vi "试剂余量显示UI.vi"() -> ()   [LabVIEW 2016, in "斯坦道总磷.lvlib"]
uses:
  <vilib>/Utility/miscctls.llb/LVPointTypeDef.ctl
panel:
  in  "余量 14":string
  in  "余量 13":string
  in  "余量 12":string
  in  "余量 11":string
  in  "余量 10":string
  in  "余量 9":string
  in  "余量 8":string
  in  "余量 7":string
  in  "余量 6":string
  in  "余量 5":string
  in  "余量 4":string
  in  "余量 3":string
  in  "余量 2":string
  in  "余量":string
  in  "关闭":bool
  in  "全部重置":bool
  in  "试剂容量设置":bool
  in  "试剂名称设置":bool
  in  "重置 14":bool
  out "试剂 14":dbl(slide) caption="V9-2.试剂14" scale=0.0..100.0 scale format="%#_f %%"
  in  "重置 13":bool
  out "试剂 13":dbl(slide) caption="V9-1.试剂13" scale=0.0..100.0 scale format="%#_f %%"
  in  "重置 12":bool
  out "试剂 12":dbl(slide) caption="V12.试剂12" scale=0.0..100.0 scale format="%#_f %%"
  in  "重置 11":bool
  out "试剂 11":dbl(slide) caption="V11.试剂11" scale=0.0..100.0 scale format="%#_f %%"
  in  "重置 10":bool
  out "试剂 10":dbl(slide) caption="V10.试剂10" scale=0.0..100.0 scale format="%#_f %%"
  in  "重置 9":bool
  out "试剂 9":dbl(slide) caption="V9.试剂9" scale=0.0..100.0 scale format="%#_f %%"
  in  "重置 8":bool
  out "试剂 8":dbl(slide) caption="V8.试剂8" scale=0.0..100.0 scale format="%#_f %%"
  in  "重置 7":bool
  out "试剂 7":dbl(slide) caption="V7.试剂7" scale=0.0..100.0 scale format="%#_f %%"
  in  "重置 6":bool
  out "试剂 6":dbl(slide) caption="V6.试剂6" scale=0.0..100.0 scale format="%#_f %%"
  in  "重置 5":bool
  out "试剂 5":dbl(slide) caption="V5.试剂5" scale=0.0..100.0 scale format="%#_f %%"
  in  "重置 4":bool
  out "试剂 4":dbl(slide) caption="V4.试剂4" scale=0.0..100.0 scale format="%#_f %%"
  in  "重置 3":bool
  out "试剂 3":dbl(slide) caption="V3.试剂3" scale=0.0..100.0 scale format="%#_f %%"
  in  "重置 2":bool
  out "试剂 2":dbl(slide) caption="V2.试剂2" scale=0.0..100.0 scale format="%#_f %%"
  in  "重置":bool
  out "试剂":dbl(slide) caption="V1.试剂1" scale=0.0..100.0 scale format="%#_f %%"
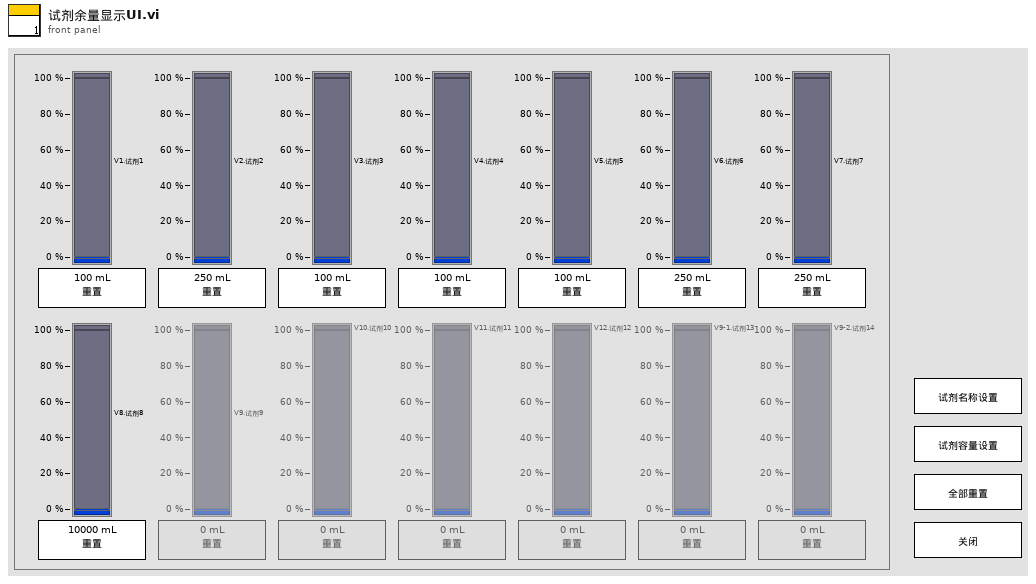
[diagram p1: front panel]
types:
  T1 = typedef "LVPointTypeDef.ctl" = cluster{"Horizontal":i16, "Vertical":i16}
  T2 = enum8{"Enabled", "Disabled", "Disabled and Grayed Out"}
  T3 = cluster{"时间标识":timestamp, "设备":string, "日志信息":string, "流程参数":string}
  T4 = cluster{"V1":sgl, "V2":sgl, "V3":sgl, "V4":sgl, "V5":sgl, "V6":sgl, "V7":sgl, "V8":sgl, "V9":sgl, "V10":sgl, "V11":sgl, "V12":sgl, "V9-1":sgl, "V9-2":sgl}
  T5 = cluster{"V":string, "V 2":string, "V 3":string, "V 4":string, "V 5":string, "V 6":string, "V 7":string, "V 8":string, "V 9":string, "V 10":string, "V 11":string, "V 12":string, "V9-1":string, "V9-2":string}
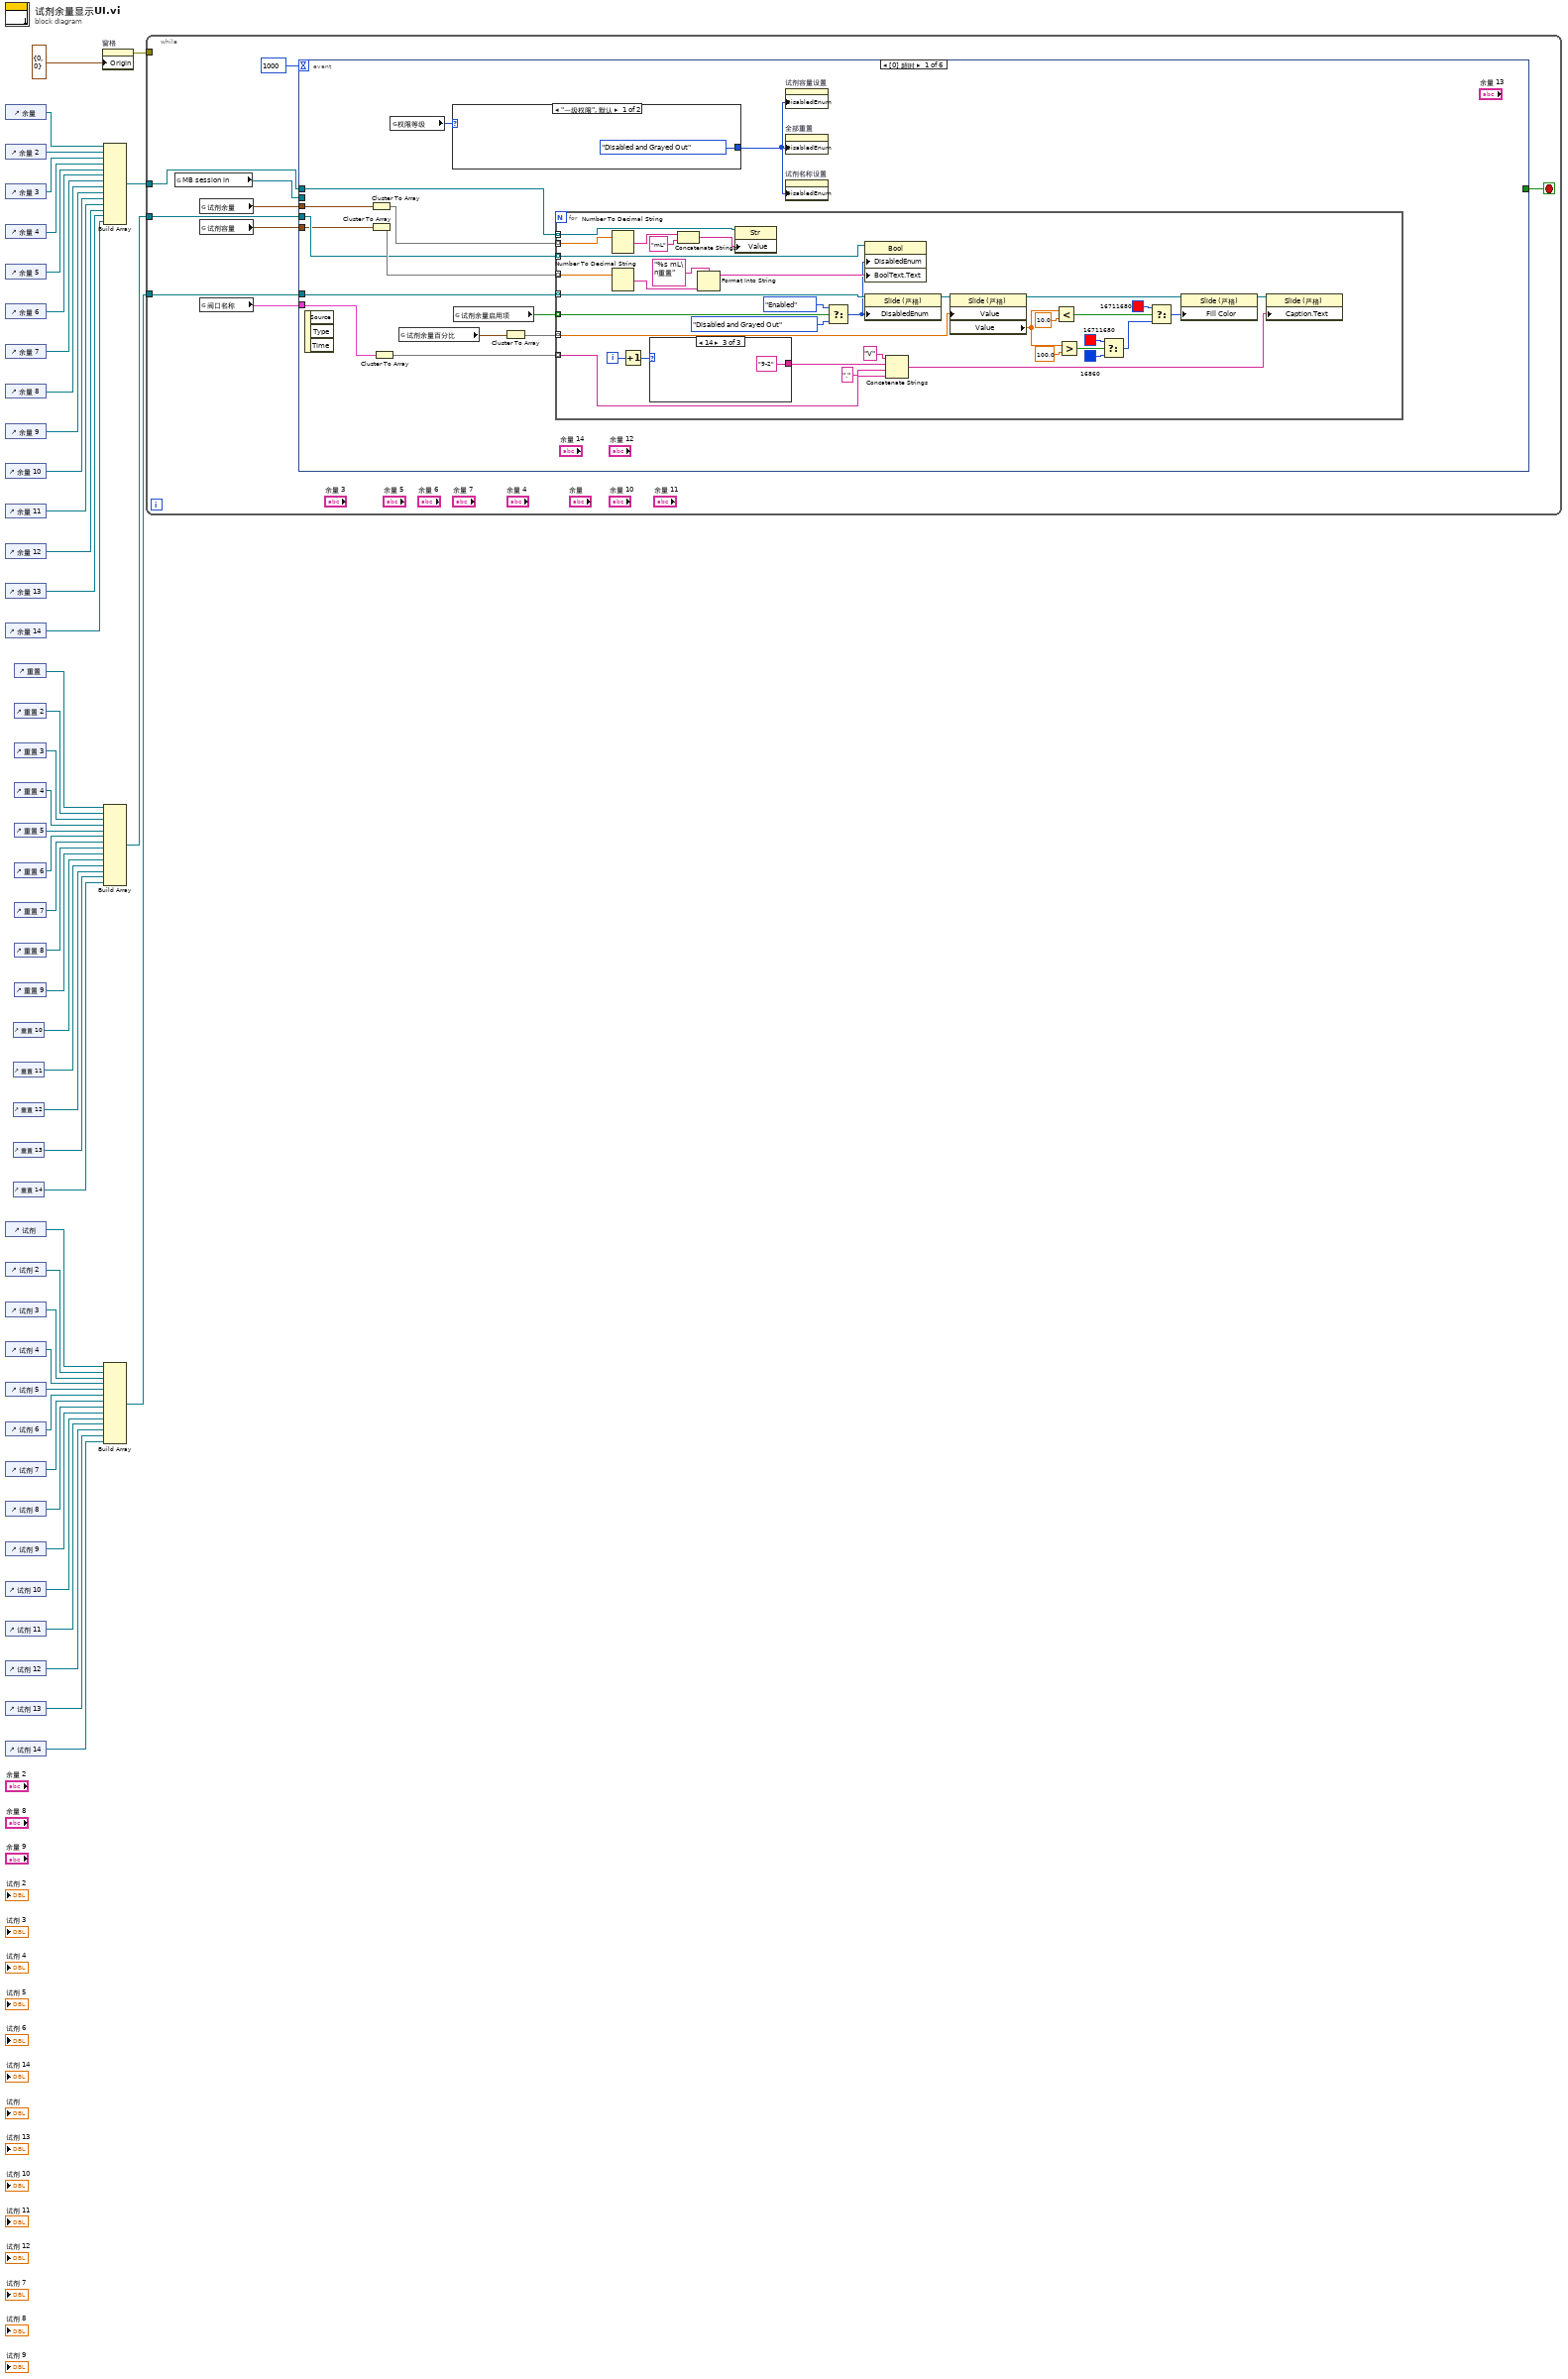
[diagram p0: block diagram]
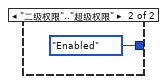
[diagram p2: hidden frame]
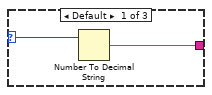
[diagram p3: hidden frame]
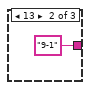
[diagram p4: hidden frame]
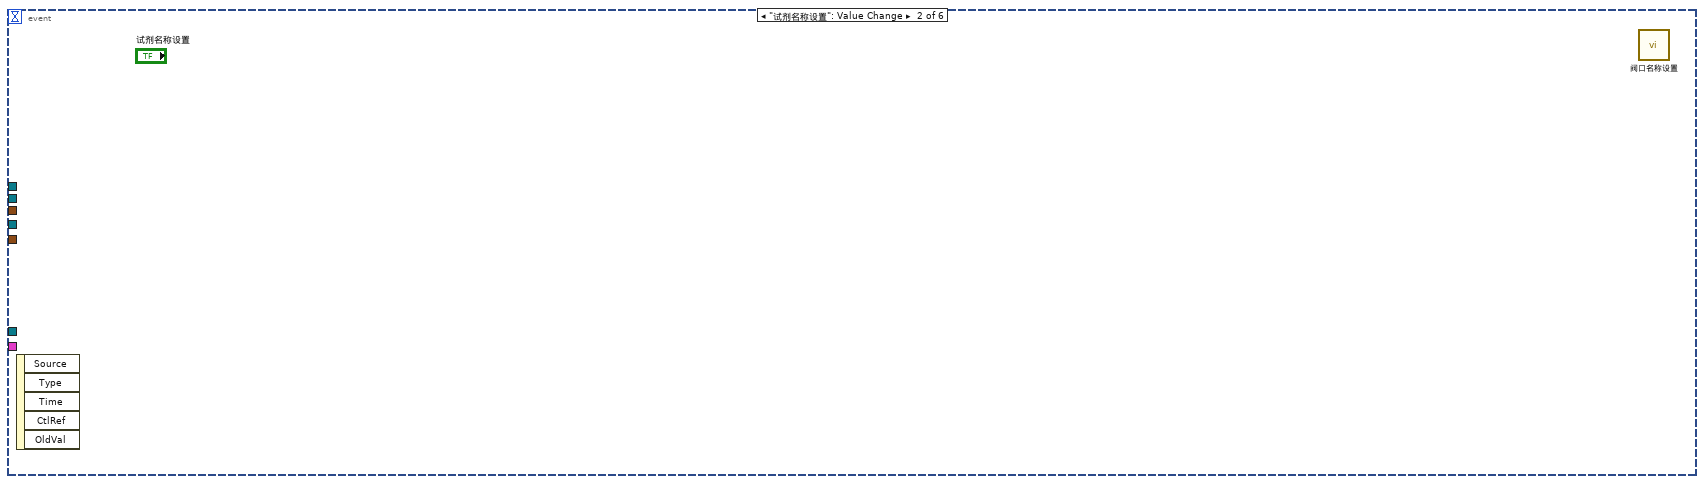
[diagram p5: hidden frame]
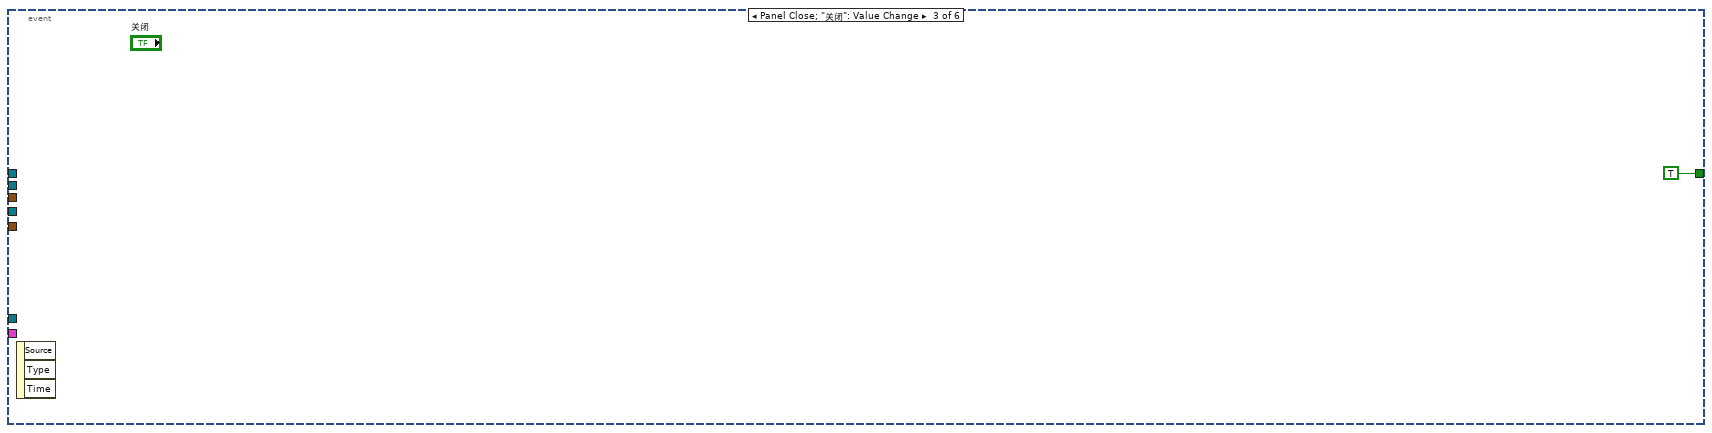
[diagram p6: hidden frame]
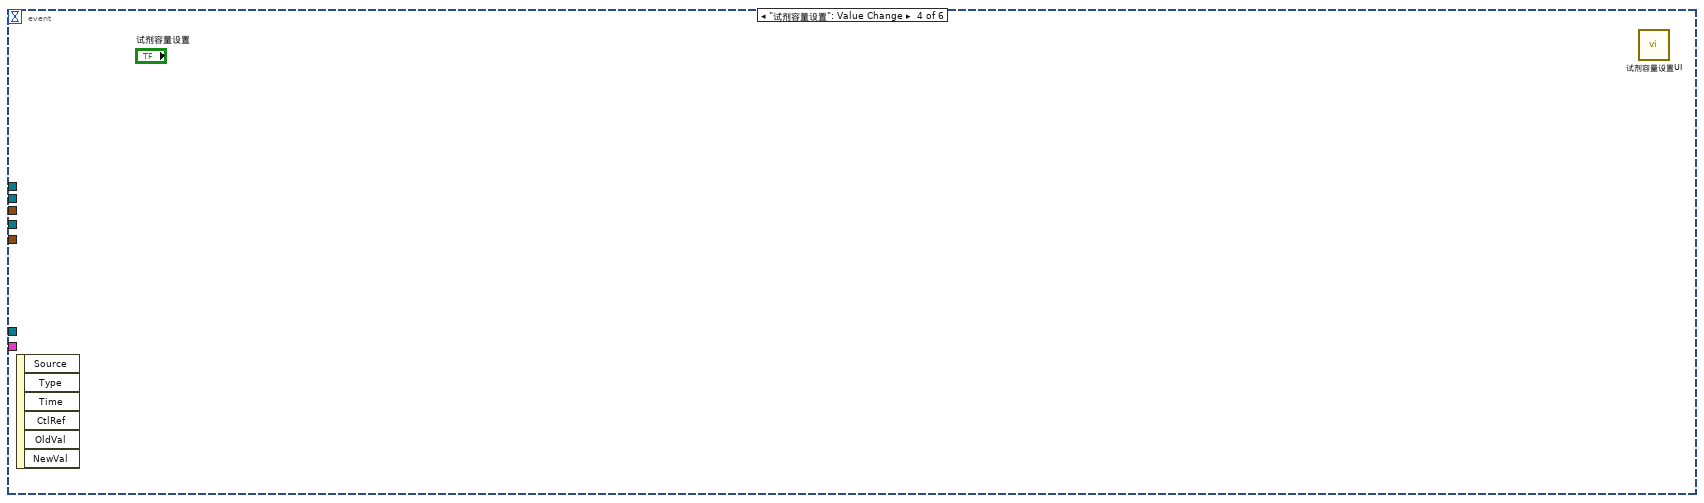
[diagram p7: hidden frame]
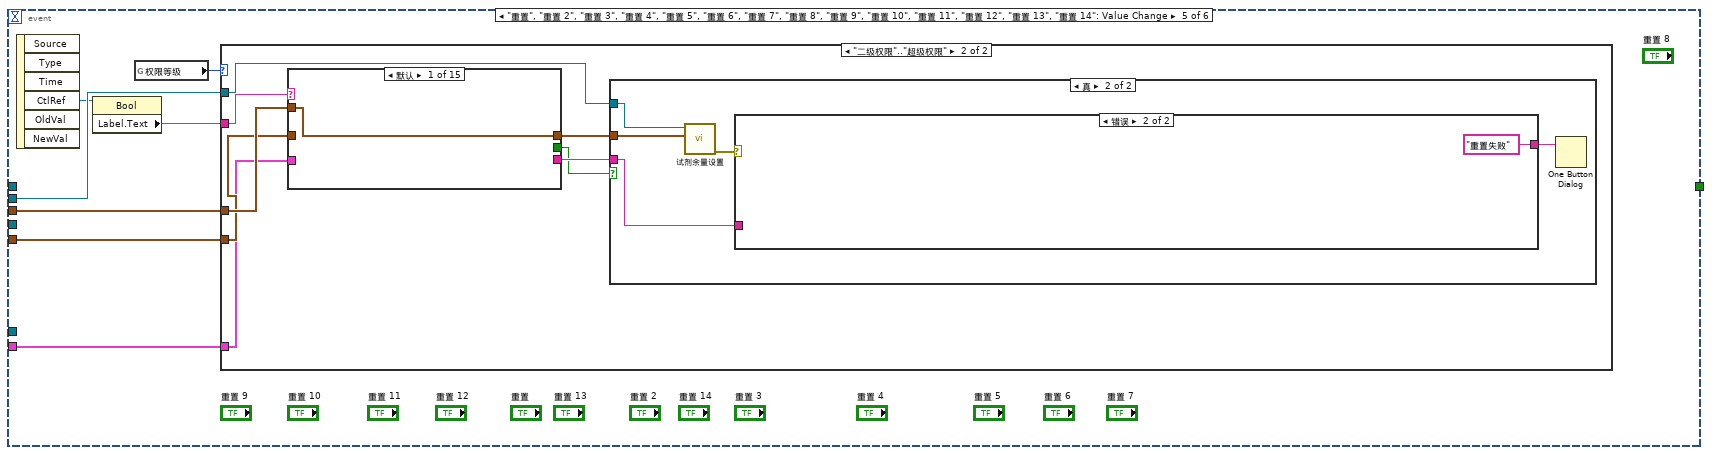
[diagram p8: hidden frame]
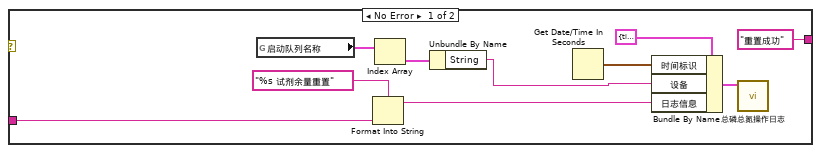
[diagram p11: hidden frame]
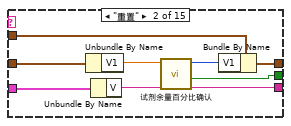
[diagram p12: hidden frame]
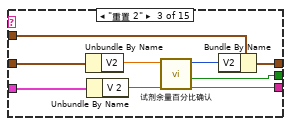
[diagram p13: hidden frame]
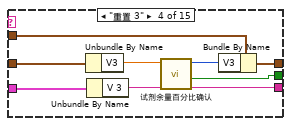
[diagram p14: hidden frame]
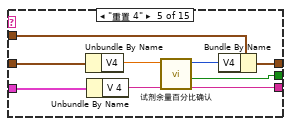
[diagram p15: hidden frame]
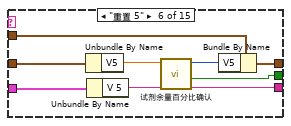
[diagram p16: hidden frame]
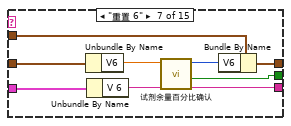
[diagram p17: hidden frame]
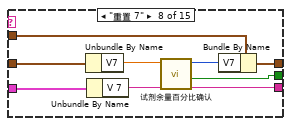
[diagram p18: hidden frame]
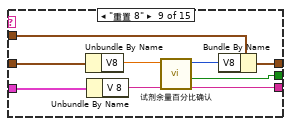
[diagram p19: hidden frame]
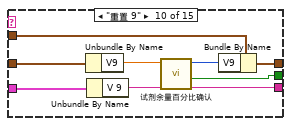
[diagram p20: hidden frame]
diagram:
  n1 = control-ref of="余量"() -> (w2:refnum<vi>)
  n2 = control-ref of="余量 2"() -> (w3:refnum<vi>)
  n3 = control-ref of="余量 3"() -> (w4:refnum<vi>)
  n4 = control-ref of="余量 4"() -> (w5:refnum<vi>)
  n5 = control-ref of="余量 5"() -> (w6:refnum<vi>)
  n6 = control-ref of="余量 6"() -> (w7:refnum<vi>)
  n7 = control-ref of="余量 7"() -> (w8:refnum<vi>)
  n8 = control-ref of="余量 8"() -> (w9:refnum<vi>)
  n9 = control-ref of="余量 9"() -> (w10:refnum<vi>)
  n10 = control-ref of="余量 10"() -> (w11:refnum<vi>)
  n11 = control-ref of="余量 11"() -> (w12:refnum<vi>)
  n12 = control-ref of="余量 12"() -> (w13:refnum<vi>)
  n13 = control-ref of="余量 13"() -> (w14:refnum<vi>)
  n14 = control-ref of="余量 14"() -> (w15:refnum<vi>)
  n15 = control-ref of="试剂"() -> (w47:refnum<vi>)
  n16 = control-ref of="试剂 2"() -> (w46:refnum<vi>)
  n17 = control-ref of="试剂 3"() -> (w45:refnum<vi>)
  n18 = control-ref of="试剂 4"() -> (w44:refnum<vi>)
  n19 = control-ref of="试剂 5"() -> (w43:refnum<vi>)
  n20 = control-ref of="试剂 6"() -> (w42:refnum<vi>)
  n21 = control-ref of="试剂 7"() -> (w41:refnum<vi>)
  n22 = control-ref of="试剂 8"() -> (w40:refnum<vi>)
  n23 = control-ref of="试剂 9"() -> (w39:refnum<vi>)
  n24 = control-ref of="试剂 10"() -> (w38:refnum<vi>)
  n25 = control-ref of="试剂 11"() -> (w37:refnum<vi>)
  n26 = control-ref of="试剂 12"() -> (w36:refnum<vi>)
  n27 = control-ref of="试剂 13"() -> (w35:refnum<vi>)
  n28 = control-ref of="试剂 14"() -> (w34:refnum<vi>)
  n29 = control-ref of="重置 10"() -> (w21:refnum<vi>)
  n30 = control-ref of="重置 11"() -> (w20:refnum<vi>)
  n31 = control-ref of="重置 12"() -> (w19:refnum<vi>)
  n32 = control-ref of="重置 13"() -> (w18:refnum<vi>)
  n33 = control-ref of="重置 14"() -> (w17:refnum<vi>)
  n34 = control-ref of="重置"() -> (w30:refnum<vi>)
  n35 = control-ref of="重置 2"() -> (w29:refnum<vi>)
  n36 = control-ref of="重置 3"() -> (w28:refnum<vi>)
  n37 = control-ref of="重置 4"() -> (w27:refnum<vi>)
  n38 = control-ref of="重置 5"() -> (w26:refnum<vi>)
  n39 = control-ref of="重置 6"() -> (w25:refnum<vi>)
  n40 = control-ref of="重置 7"() -> (w24:refnum<vi>)
  n41 = control-ref of="重置 8"() -> (w23:refnum<vi>)
  n42 = control-ref of="重置 9"() -> (w22:refnum<vi>)
  n43 = property on="窗格" class="Pane"("Origin"=T1 {"Horizontal"=0, "Vertical"=0} ("原点")) -> (error out=w31:errorcluster)  [unwired: 2 in, 1 out]
  n44 = Build Array(w2, w3, w4, w5, w6, w7, w8, w9, w10, w11, w12, w13, w14, w15) -> (w1:refnum<vi>[])
  n45 = Build Array(w30, w29, w28, w27, w26, w25, w24, w23, w22, w21, w20, w19, w18, w17) -> (w16:refnum<vi>[])
  n46 = Build Array(w47, w46, w45, w44, w43, w42, w41, w40, w39, w38, w37, w36, w35, w34) -> (w33:refnum<vi>[])
  n47 = while {
    tunnel: w33 -> [w56]
    tunnel: w31 -> [_]
    tunnel: w16 -> [w55]
    tunnel: w1 -> [w51]
    stop <- w54 stop-if-true
    n48 = global read "VAR总磷总氮全局变量.vi" "MB session in"() -> (w52:refnum<class "MB_Master.lvclass">)
    n49 = global read "VAR总磷总氮全局变量.vi" "试剂余量"() -> (w49:T4)
    n50 = global read "VAR总磷总氮全局变量.vi" "试剂容量"() -> (w50:T4)
    n51 = global read "总磷总氮断电保存全局变量.vi" "阀口名称"() -> (w48:T5)
    n52 = event shown="[0] 超时" {
      selector: _ -> [_ _ _ _ _ _]
      dyn-events: _ -> [_ _ _ _ _ _]
      timeout: 1000 -> [_ _ _ _ _ _]
      tunnel: w56 -> [w70 _ _ _ _ _]
      tunnel: w55 -> [w67 _ _ _ _ _]
      tunnel: [_ _ TRUE _ _ _] -> w54
      tunnel: w50 -> [w61 _ _ _ w116 _]
      tunnel: w49 -> [w60 _ _ _ w119 _]
      tunnel: w52 -> [_ _ _ _ w120 w259]
      tunnel: w51 -> [w64 _ _ _ _ _]
      tunnel: w48 -> [w57 _ _ _ w114 _]
      event Timeout {
        n53 = event-data() -> ()  [unwired: 1 in, 3 out]
        n54 = Cluster To Array(cluster=w60) -> (array=w65:sgl[])
        n55 = Cluster To Array(cluster=w61) -> (array=w68:sgl[])
        n56 = Cluster To Array(cluster=w57) -> (array=w66:string[])
        n57 = global read "VAR总磷总氮全局变量.vi" "权限等级"() -> (w59:enum16{"一级权限", "二级权限", "三级权限", "超级权限"})
        n58 = global read "VAR总磷总氮全局变量.vi" "试剂余量百分比"() -> (w62:T4)
        n59 = case shown="\"一级权限\", 默认" w59 {
          tunnel: [T2."Disabled and Grayed Out" ("禁用") T2."Enabled" ("禁用")] -> w58
          frame "一级权限", Default {
          }
          frame "二级权限".."超级权限" {
          }
        }
        n60 = global read "VAR总磷总氮全局变量.vi" "试剂余量启用项"() -> (w63:bool[])
        n61 = Cluster To Array(cluster=w62) -> (array=w69:sgl[])
        n62 = for {
          tunnel: w70 -> [w102] mode=indexing
          tunnel: w69 -> [w103] mode=indexing
          tunnel: w68 -> [w91] mode=indexing
          tunnel: w67 -> [w100] mode=indexing
          tunnel: w66 -> [w97] mode=indexing
          tunnel: w65 -> [w87] mode=indexing
          tunnel: w64 -> [w86] mode=indexing
          tunnel: w63 -> [w82] mode=indexing
          i -> [w94]
          n63 = Number To Decimal String(number=w87) -> (decimal integer string=w85:string)  [unwired: 1 in]
          n64 = Number To Decimal String(number=w91) -> (decimal integer string=w90:string)  [unwired: 1 in]
          n65 = Increment(x=w94) -> (x+1=w93:i32)
          n66 = case shown="14" w93 {
            selector: w93 -> [w110 _ _]
            tunnel: [w109 "9-1" "9-2"] -> w92
            frame Default {
              n67 = Number To Decimal String(number=w110) -> (decimal integer string=w109:string)  [unwired: 1 in]
            }
            frame 13 {
            }
            frame 14 {
            }
          }
          n68 = Concatenate Strings(w85, "mL" ("字符串")) -> (w84:string)
          n69 = Format Into String(format string="%s mL\n重置" ("格式字符串"), w90) -> (resulting string=w88:string)  [unwired: 2 in, 1 out]
          n70 = property class="Str"(reference=w86, "Value"=w84) -> ()  [unwired: 1 in, 2 out]
          n71 = Select(t=T2."Enabled" ("禁用"), s=w82, f=T2."Disabled and Grayed Out" ("禁用")) -> (s? t:f=w81:T2)
          n72 = property class="Bool"(reference=w100, "DisabledEnum"=w81, "BoolText.Text"=w88) -> ()  [unwired: 1 in, 2 out]
          n73 = property class="Slide (严格)"(reference=w102, "DisabledEnum"=w81) -> (reference out=w101:refnum<vi>)  [unwired: 1 in, 1 out]
          n74 = Concatenate Strings("V" ("字符串"), w92, "." ("字符串"), w97) -> (w96:string)
          n75 = property class="Slide (严格)"(reference=w101, "Value"=w103) -> (reference out=w107:refnum<vi>, "Value"=w78:dbl)  [unwired: 1 in, 1 out]
          n76 = Less?(x=w78, y=10.0) -> (x < y?=w106:bool)
          n77 = Greater?(x=w78, y=100.0) -> (0:w76:bool)
          n78 = Select(t=u32 16711680 ("滑块颜色:背景色"), s=w76, f=u32 16860 ("滑块颜色:背景色")) -> (s? t:f=w73:u32)
          n79 = Select(t=u32 16711680 ("滑块颜色:背景色"), s=w106, f=w73) -> (s? t:f=w104:u32)
          n80 = property class="Slide (严格)"(reference=w107, "Fill Color"=w104) -> (reference out=w99:refnum<vi>)  [unwired: 1 in, 1 out]
          n81 = property class="Slide (严格)"(reference=w99, "Caption.Text"=w96) -> ()  [unwired: 1 in, 2 out]
        }
        n82 = property on="试剂容量设置" class="Bool"("DisabledEnum"=w58) -> ()  [unwired: 2 in, 2 out]
        n83 = property on="全部重置" class="Bool"("DisabledEnum"=w58) -> ()  [unwired: 2 in, 2 out]
        n84 = property on="试剂名称设置" class="Bool"("DisabledEnum"=w58) -> ()  [unwired: 2 in, 2 out]
      }
      event "试剂名称设置": Value Change {
        n85 = event-data() -> ()  [unwired: 1 in, 5 out]
        n86 = call "阀口名称设置.vi"() -> ()  [unwired: 12 in]
      }
      event Panel Close; "关闭": Value Change {
        n87 = event-data() -> ()  [unwired: 1 in, 3 out]
      }
      event "试剂容量设置": Value Change {
        n88 = event-data() -> ()  [unwired: 1 in, 6 out]
        n89 = call "试剂容量设置UI.vi"() -> ()  [unwired: 12 in]
      }
      event "重置", "重置 2", "重置 3", "重置 4", "重置 5", "重置 6", "重置 7", "重置 8", "重置 9", "重置 10", "重置 11", "重置 12", "重置 13", "重置 14": Value Change {
        n90 = event-data() -> ("CtlRef"=w118:refnum<vi>)  [unwired: 1 in, 5 out]
        n91 = property class="Bool"(reference=w118) -> ("Label.Text"=w117:string)  [unwired: 1 in, 2 out]
        n92 = global read "VAR总磷总氮全局变量.vi" "权限等级"() -> (w115:enum16{"一级权限", "二级权限", "三级权限", "超级权限"})
        n93 = case shown="\"二级权限\"..\"超级权限\"" w115 {
          tunnel: w120 -> [_ w128]
          tunnel: w119 -> [_ w127]
          tunnel: w117 -> [_ w125]
          tunnel: w116 -> [_ w124]
          tunnel: w114 -> [_ w123]
          frame "一级权限", Default {
          }
          frame "二级权限".."超级权限" {
            n94 = case shown="默认" w125 {
              tunnel: w127 -> [w145 w153 w161 w169 w177 w185 w193 w201 w209 w217 w225 w233 w241 w249 w257]
              tunnel: [w145 w152 w160 w168 w176 w184 w192 w200 w208 w216 w224 w232 w240 w248 w256] -> w126
              tunnel: w124 -> [_ w151 w159 w167 w175 w183 w191 w199 w207 w215 w223 w231 w239 w247 w255]
              tunnel: w123 -> [_ w148 w156 w164 w172 w180 w188 w196 w204 w212 w220 w228 w236 w244 w252]
              tunnel: [_ w147 w155 w163 w171 w179 w187 w195 w203 w211 w219 w227 w235 w243 w251] -> w122
              tunnel: [_ w146 w154 w162 w170 w178 w186 w194 w202 w210 w218 w226 w234 w242 w250] -> w121
              frame Default {
              }
              frame "重置" {
                n95 = Unbundle By Name(w151) -> ("V1"=w150:sgl)
                n96 = Unbundle By Name(w148) -> ("V"=w147:string)
                n97 = call "试剂余量百分比确认.vi"("试剂余量百分比 2"=w150) -> ("Value"=w149:u16, "check ？"=w146:bool)  [unwired: 9 in]
                n98 = Bundle By Name(cluster=w153, "V1"=w149) -> (w152:T4)
              }
              frame "重置 2" {
                n99 = Unbundle By Name(w159) -> ("V2"=w158:sgl)
                n100 = Unbundle By Name(w156) -> ("V 2"=w155:string)
                n101 = call "试剂余量百分比确认.vi"("试剂余量百分比 2"=w158) -> ("Value"=w157:u16, "check ？"=w154:bool)  [unwired: 9 in]
                n102 = Bundle By Name(cluster=w161, "V2"=w157) -> (w160:T4)
              }
              frame "重置 3" {
                n103 = Unbundle By Name(w167) -> ("V3"=w166:sgl)
                n104 = Unbundle By Name(w164) -> ("V 3"=w163:string)
                n105 = call "试剂余量百分比确认.vi"("试剂余量百分比 2"=w166) -> ("Value"=w165:u16, "check ？"=w162:bool)  [unwired: 9 in]
                n106 = Bundle By Name(cluster=w169, "V3"=w165) -> (w168:T4)
              }
              frame "重置 4" {
                n107 = Unbundle By Name(w175) -> ("V4"=w174:sgl)
                n108 = Unbundle By Name(w172) -> ("V 4"=w171:string)
                n109 = call "试剂余量百分比确认.vi"("试剂余量百分比 2"=w174) -> ("Value"=w173:u16, "check ？"=w170:bool)  [unwired: 9 in]
                n110 = Bundle By Name(cluster=w177, "V4"=w173) -> (w176:T4)
              }
              frame "重置 5" {
                n111 = Unbundle By Name(w183) -> ("V5"=w182:sgl)
                n112 = Unbundle By Name(w180) -> ("V 5"=w179:string)
                n113 = call "试剂余量百分比确认.vi"("试剂余量百分比 2"=w182) -> ("Value"=w181:u16, "check ？"=w178:bool)  [unwired: 9 in]
                n114 = Bundle By Name(cluster=w185, "V5"=w181) -> (w184:T4)
              }
              frame "重置 6" {
                n115 = Unbundle By Name(w191) -> ("V6"=w190:sgl)
                n116 = Unbundle By Name(w188) -> ("V 6"=w187:string)
                n117 = call "试剂余量百分比确认.vi"("试剂余量百分比 2"=w190) -> ("Value"=w189:u16, "check ？"=w186:bool)  [unwired: 9 in]
                n118 = Bundle By Name(cluster=w193, "V6"=w189) -> (w192:T4)
              }
              frame "重置 7" {
                n119 = Unbundle By Name(w199) -> ("V7"=w198:sgl)
                n120 = Unbundle By Name(w196) -> ("V 7"=w195:string)
                n121 = call "试剂余量百分比确认.vi"("试剂余量百分比 2"=w198) -> ("Value"=w197:u16, "check ？"=w194:bool)  [unwired: 9 in]
                n122 = Bundle By Name(cluster=w201, "V7"=w197) -> (w200:T4)
              }
              frame "重置 8" {
                n123 = Unbundle By Name(w207) -> ("V8"=w206:sgl)
                n124 = Unbundle By Name(w204) -> ("V 8"=w203:string)
                n125 = call "试剂余量百分比确认.vi"("试剂余量百分比 2"=w206) -> ("Value"=w205:u16, "check ？"=w202:bool)  [unwired: 9 in]
                n126 = Bundle By Name(cluster=w209, "V8"=w205) -> (w208:T4)
              }
              frame "重置 9" {
                n127 = Unbundle By Name(w215) -> ("V9"=w214:sgl)
                n128 = Unbundle By Name(w212) -> ("V 9"=w211:string)
                n129 = call "试剂余量百分比确认.vi"("试剂余量百分比 2"=w214) -> ("Value"=w213:u16, "check ？"=w210:bool)  [unwired: 9 in]
                n130 = Bundle By Name(cluster=w217, "V9"=w213) -> (w216:T4)
              }
              frame "重置 10" {
                n131 = Unbundle By Name(w220) -> ("V 10"=w219:string)
                n132 = Unbundle By Name(w223) -> ("V10"=w222:sgl)
                n133 = call "试剂余量百分比确认.vi"("试剂余量百分比 2"=w222) -> ("Value"=w221:u16, "check ？"=w218:bool)  [unwired: 9 in]
                n134 = Bundle By Name(cluster=w225, "V10"=w221) -> (w224:T4)
              }
              frame "重置 11" {
                n135 = Unbundle By Name(w228) -> ("V 11"=w227:string)
                n136 = Unbundle By Name(w231) -> ("V11"=w230:sgl)
                n137 = call "试剂余量百分比确认.vi"("试剂余量百分比 2"=w230) -> ("Value"=w229:u16, "check ？"=w226:bool)  [unwired: 9 in]
                n138 = Bundle By Name(cluster=w233, "V11"=w229) -> (w232:T4)
              }
              frame "重置 12" {
                n139 = Unbundle By Name(w236) -> ("V 12"=w235:string)
                n140 = Unbundle By Name(w239) -> ("V12"=w238:sgl)
                n141 = call "试剂余量百分比确认.vi"("试剂余量百分比 2"=w238) -> ("Value"=w237:u16, "check ？"=w234:bool)  [unwired: 9 in]
                n142 = Bundle By Name(cluster=w241, "V12"=w237) -> (w240:T4)
              }
              frame "重置 13" {
                n143 = Unbundle By Name(w247) -> ("V9-1"=w246:sgl)
                n144 = Unbundle By Name(w244) -> ("V9-1"=w243:string)
                n145 = call "试剂余量百分比确认.vi"("试剂余量百分比 2"=w246) -> ("Value"=w245:u16, "check ？"=w242:bool)  [unwired: 9 in]
                n146 = Bundle By Name(cluster=w249, "V9-1"=w245) -> (w248:T4)
              }
              frame "重置 14" {
                n147 = Unbundle By Name(w255) -> ("V9-2"=w254:sgl)
                n148 = Unbundle By Name(w252) -> ("V9-2"=w251:string)
                n149 = call "试剂余量百分比确认.vi"("试剂余量百分比 2"=w254) -> ("Value"=w253:u16, "check ？"=w250:bool)  [unwired: 9 in]
                n150 = Bundle By Name(cluster=w257, "V9-2"=w253) -> (w256:T4)
              }
            }
            n151 = case shown="真" w121 {
              tunnel: w128 -> [_ w133]
              tunnel: w126 -> [_ w132]
              tunnel: w122 -> [_ w129]
              frame False {
              }
              frame True {
                n152 = call "试剂余量设置.vi"("试剂余量"=w132, "MB session in"=w133) -> ("error out"=w131:errorcluster)  [unwired: 8 in, 1 out]
                n153 = case shown="错误" w131 {
                  tunnel: ["重置成功" ("消息") "重置失败" ("消息")] -> w130
                  tunnel: w129 -> [w136 _]
                  frame No Error {
                    n154 = global read "总磷总氮断电保存全局变量.vi" "启动队列名称"() -> (w140:cluster{"String":string, "Value":u16}[])
                    n155 = Format Into String(format string="%s 试剂余量重置" ("格式字符串"), w136) -> (resulting string=w134:string)  [unwired: 2 in, 1 out]
                    n156 = Index Array(array=w140) -> (element=w141:cluster{"String":string, "Value":u16})  [unwired: 1 in]
                    n157 = Unbundle By Name(w141) -> ("String"=w142:string)
                    n158 = Get Date/Time In Seconds() -> (seconds since 1Jan1904=w139:timestamp)
                    n159 = Bundle By Name(cluster=T3 {"时间标识"=timestamp(0 s since 1904-01-01), "设备"="", "日志信息"="", "流程参数"=""} ("data in"), "时间标识"=w139, "设备"=w142, "日志信息"=w134) -> (w138:T3)
                    n160 = call "总磷总氮操作日志.vi"("data in"=w138) -> ()  [unwired: 11 in]
                  }
                  frame Error {
                  }
                }
                n161 = One Button Dialog(message=w130) -> ()  [unwired: 1 in, 1 out]
              }
            }
          }
        }
      }
      event "全部重置": Value Change {
        n162 = event-data() -> ()  [unwired: 1 in, 6 out]
        n163 = global read "VAR总磷总氮全局变量.vi" "权限等级"() -> (w258:enum16{"一级权限", "二级权限", "三级权限", "超级权限"})
        n164 = case shown="\"二级权限\"..\"超级权限\"" w258 {
          tunnel: w259 -> [_ w262]
          frame "一级权限", Default {
          }
          frame "二级权限".."超级权限" {
            n165 = call "试剂余量重置.vi"("MB session in"=w262) -> ("error out"=w260:errorcluster)  [unwired: 9 in, 1 out]
            n166 = case shown="错误" w260 {
              tunnel: ["重置成功" ("消息") "重置失败" ("消息")] -> w261
              frame No Error {
              }
              frame Error {
              }
            }
            n167 = One Button Dialog(message=w261) -> ()  [unwired: 1 in, 1 out]
          }
        }
      }
    }
  }
